vi "main.vi"() -> ()   [LabVIEW 2018]
uses:
  Module/User Event/User Event.lvlib
  Module/Message Queue/Message Queue.lvlib
  Module/Message Queue/Enqueue Message (Single).vi
  UI/TypeDefine/EnumMainDlgInit.ctl
  MainUIRef.ctl
  Module/Library-Ctrl/Library-Ctrl.lvlib
panel:
  in  "선택항목 모든버전 삭제 버튼":bool
  in  "선택항목 삭제 버튼":bool
  in  "업로드버튼":bool
  in  "업로드할 파일 정보 입력란":T1
  in  "main-lstDetailFileInfo":i32(listbox)
  in  "main-lstFileList":i32(listbox)
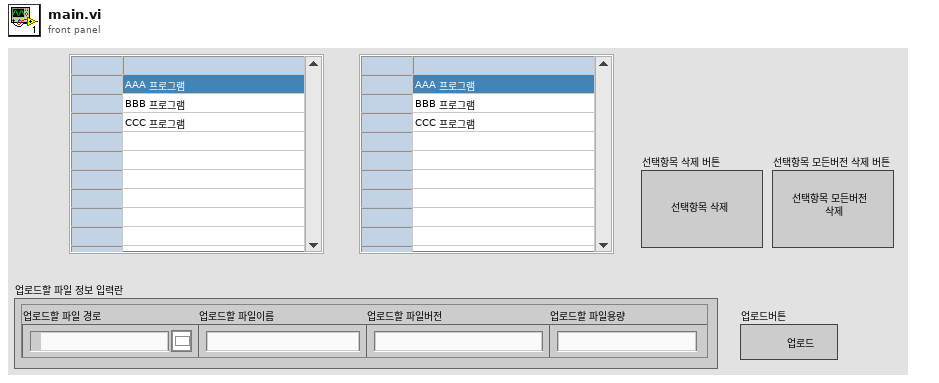
[diagram p1: front panel]
types:
  T1 = cluster{"업로드할 파일 경로":path, "업로드할 파일이름":string, "업로드할 파일버전":string, "업로드할 파일용량":string}
  T2 = typedef "MainUIRef.ctl" = cluster{"btn":cluster{"bStartBtn":refnum<vi>, "bStopBtn":refnum<vi>, "bReportBtn":refnum<vi>, "bUnitStartBtn":refnum<vi>, "bScanBtn":refnum<vi>, "bSettingBtn":refnum<vi>, "bRepeatBtn":refnum<vi>}, "status":cluster{"bEnableFailStop":refnum<vi>, "bEnableSafety":refnum<vi>, "bTestRunCheck":refnum<vi>, "bIsCompletedMaster":refnum<vi>}, "main":cluster{"lstFileList":refnum<vi>, "lstDetailFileInfo":refnum<vi>}}
  T3 = cluster{"MainUIRef":T2, "User Event":refnum<user-event>}
  T4 = cluster{"bStartBtn":refnum<vi>, "bStopBtn":refnum<vi>, "bReportBtn":refnum<vi>, "bUnitStartBtn":refnum<vi>, "bScanBtn":refnum<vi>, "bSettingBtn":refnum<vi>, "bRepeatBtn":refnum<vi>}
  T5 = cluster{"bEnableFailStop":refnum<vi>, "bEnableSafety":refnum<vi>, "bTestRunCheck":refnum<vi>, "bIsCompletedMaster":refnum<vi>}
  T6 = cluster{"lstFileList":refnum<vi>, "lstDetailFileInfo":refnum<vi>}
  T7 = typedef "Message Queue.lvlib/All Message Queues.ctl" = cluster{"UI":refnum<queue>, "Display":refnum<queue>, "Timer":refnum<queue>}
  T8 = typedef "EnumMainDlgInit.ctl" = enum16{"start", "initRef", "InitDisplayUI", "InitSetting", "InitModule", "InitOperation", "SetuipDisplayUI", "end"}
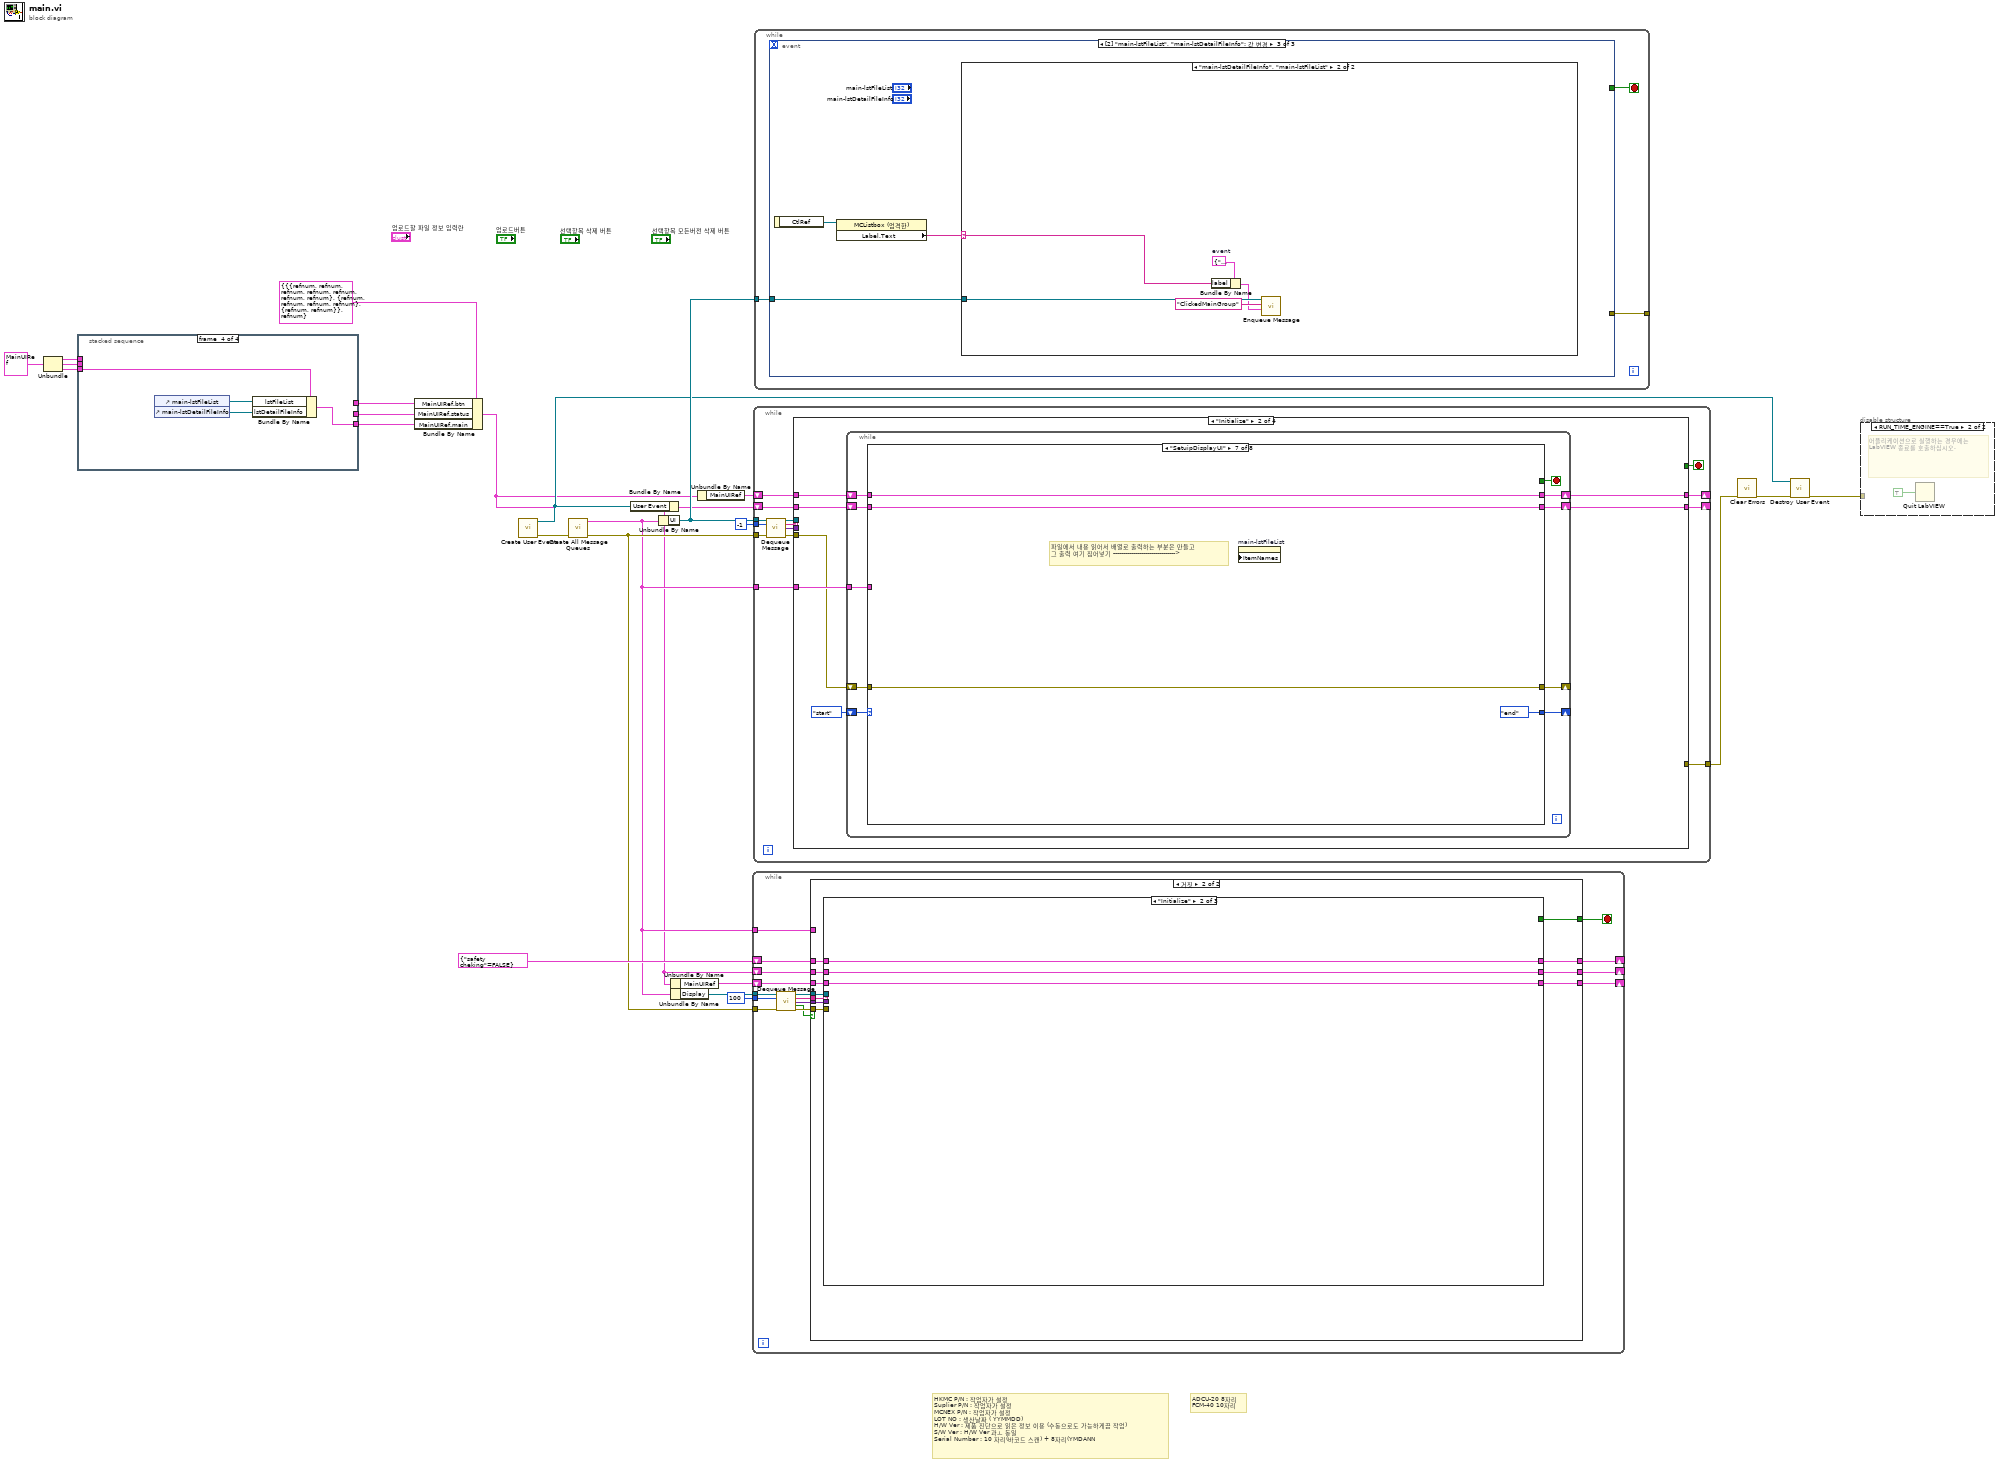
[diagram p0: block diagram]
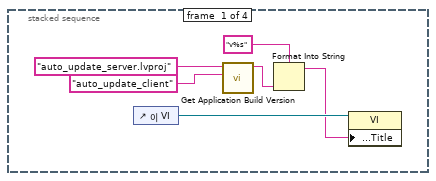
[diagram p2: hidden frame]
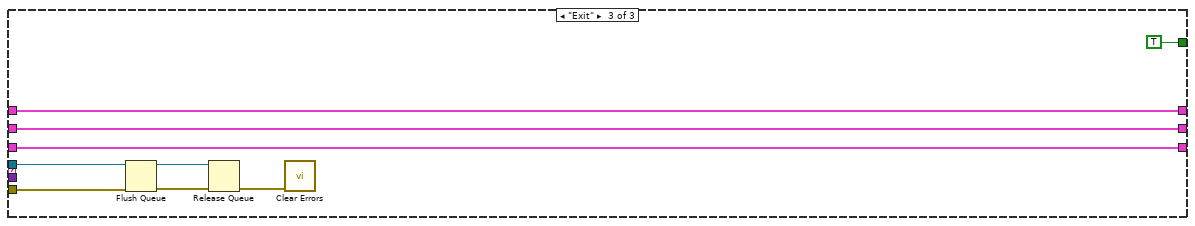
[diagram p8: hidden frame]
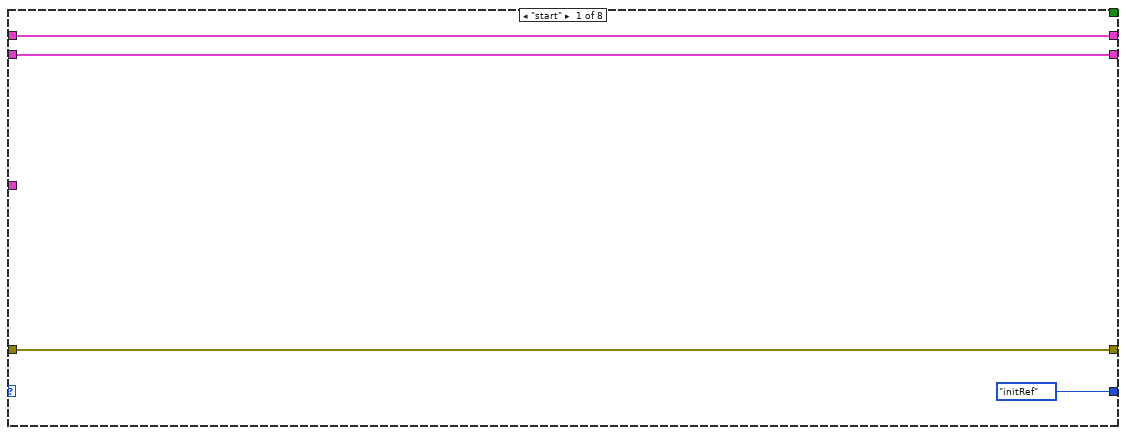
[diagram p10: hidden frame]
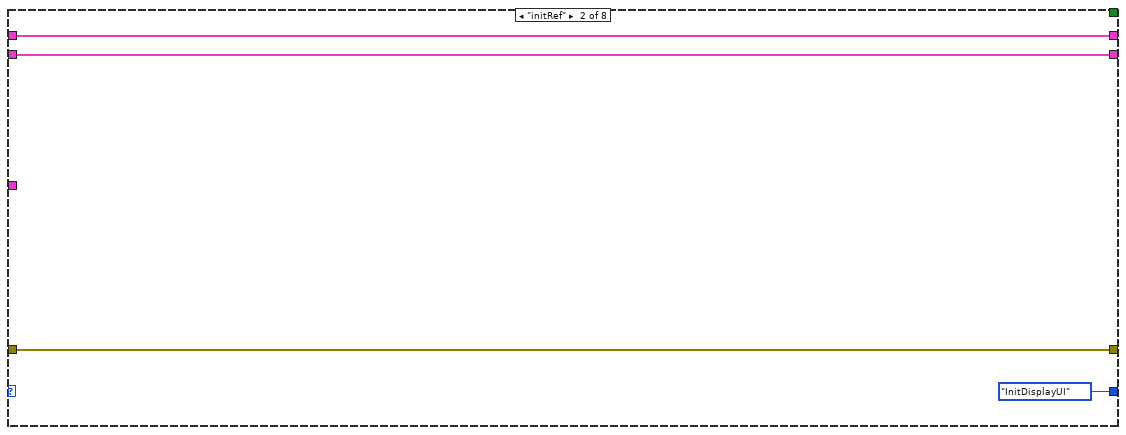
[diagram p11: hidden frame]
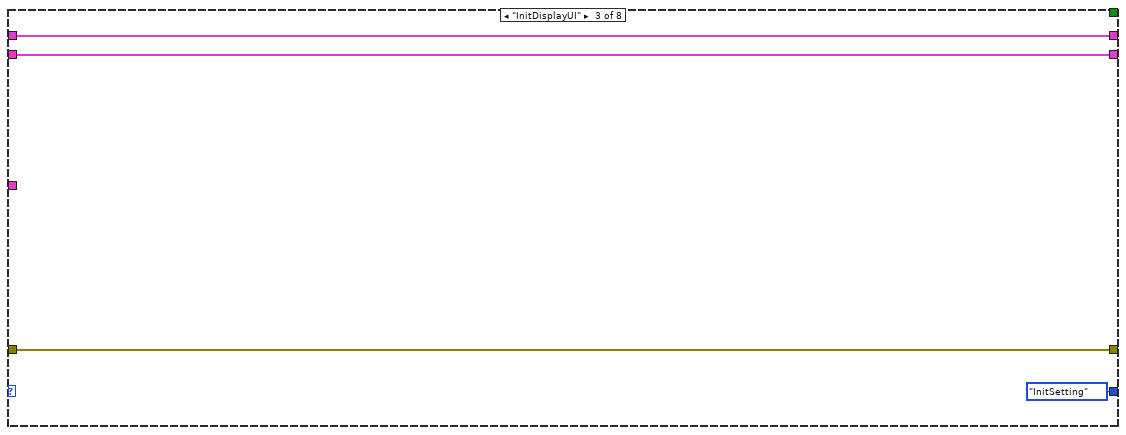
[diagram p12: hidden frame]
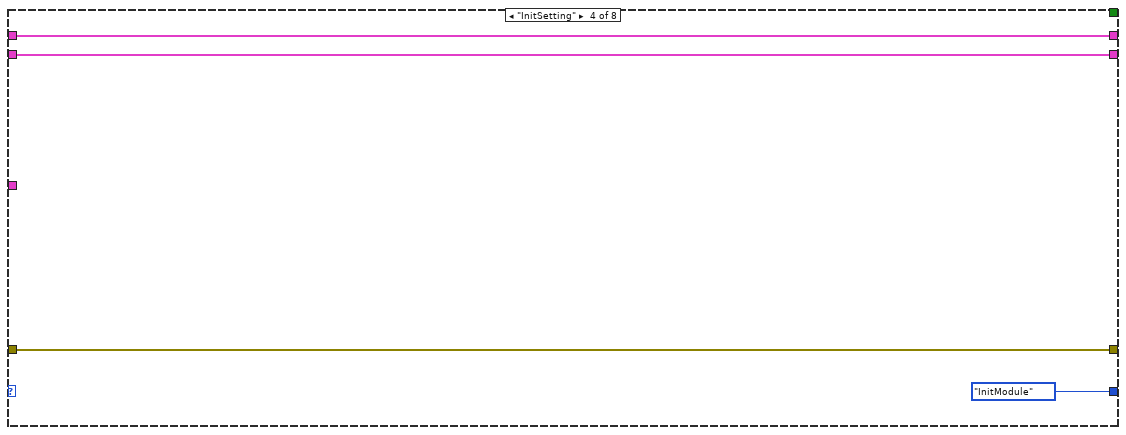
[diagram p13: hidden frame]
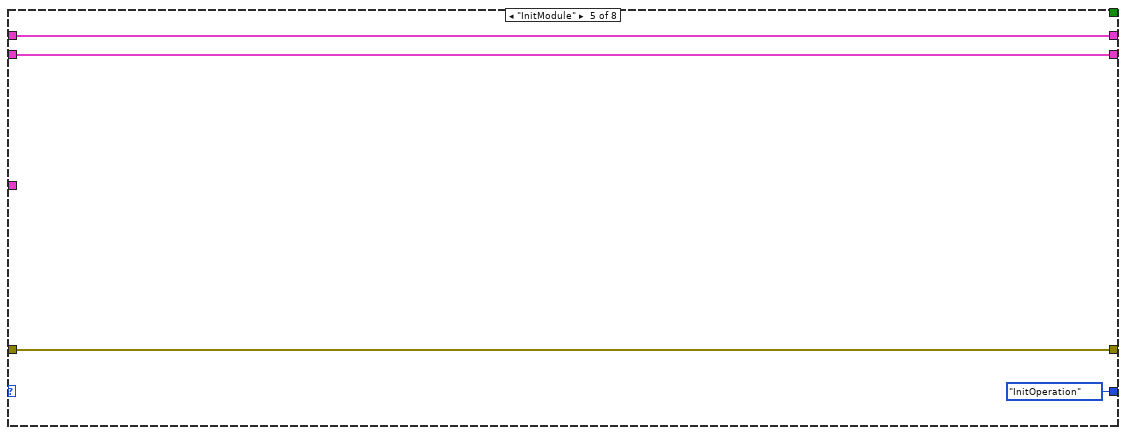
[diagram p14: hidden frame]
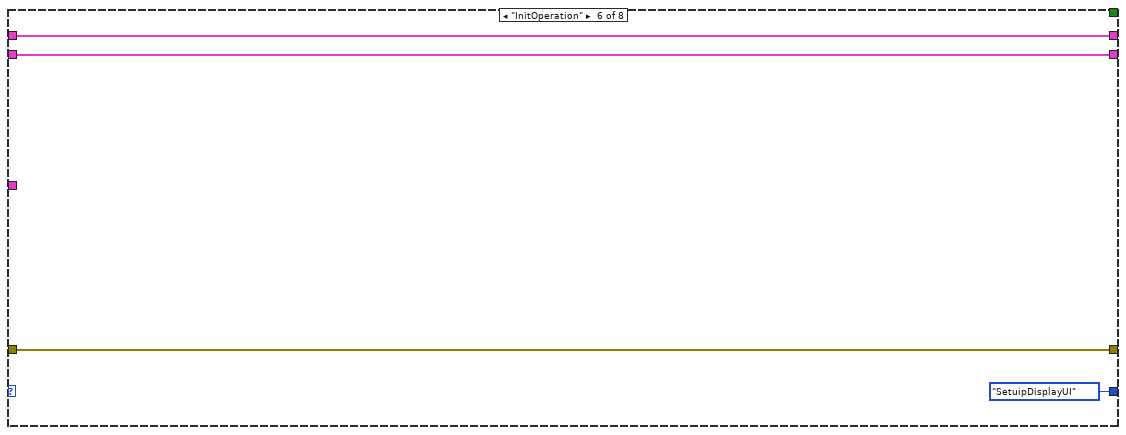
[diagram p15: hidden frame]
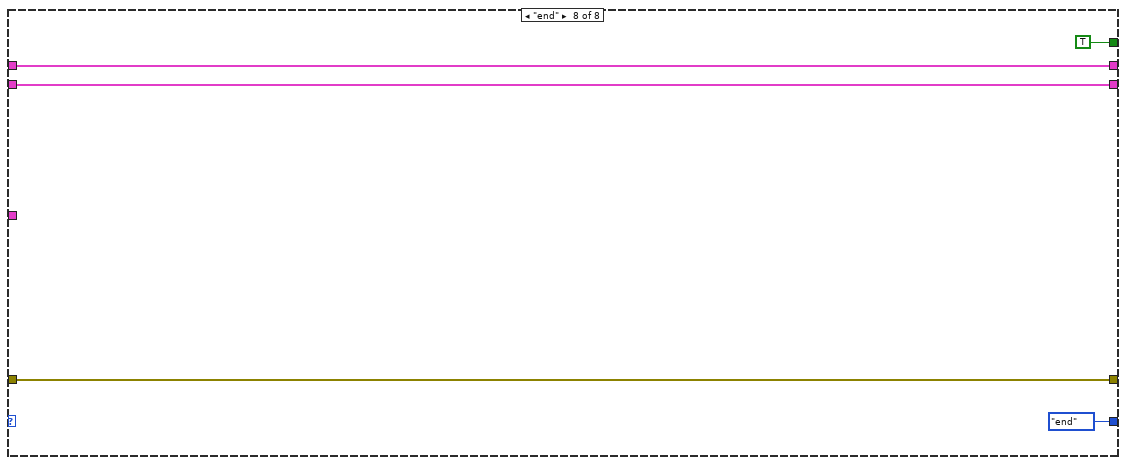
[diagram p16: hidden frame]
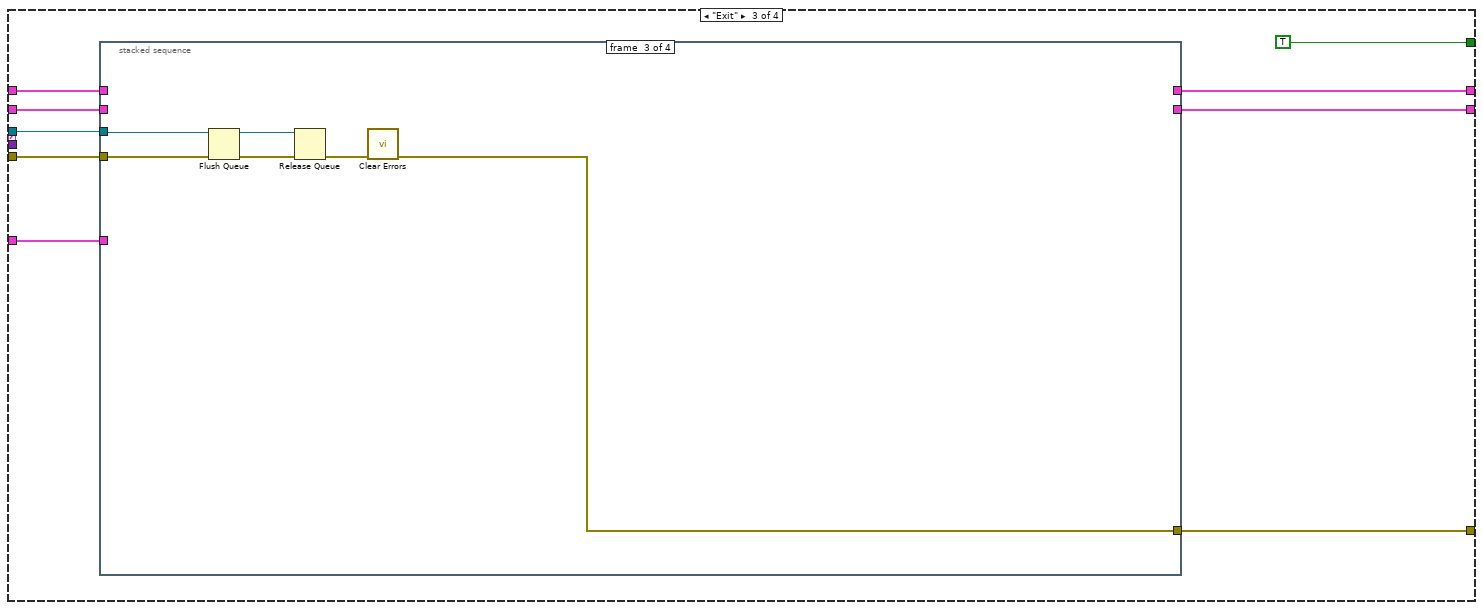
[diagram p17: hidden frame]
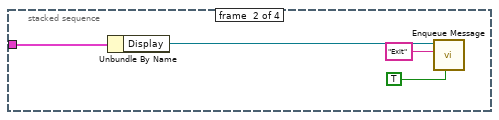
[diagram p19: hidden frame]
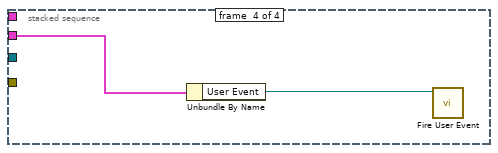
[diagram p20: hidden frame]
diagram:
  # "ADCU-20 8자리\nFCM-40 10자리"
  # "HKMC P/N : 작업자가 설정\nSuplier P/N : 작업자가 설정\nMCNEX P/N : 작업자가 설정\nLOT NO : 생산날짜 ( YYMMDD)\nH/W Ver : 제품 진단으로 읽은 정보 이용 (수동으로도 가능하게끔 작업)\nS/W Ver : H/W Ver 과ㅗ 동일\nSerial Number : 10 자리(바코드 스캔) + 8자리(YMDANN"
  n1 = Unbundle(T2 {"btn"={"bStartBtn"=refnum, "bStopBtn"=refnum, "bReportBtn"=refnum, "bUnitStartBtn"=refnum, "bScanBtn"=refnum, "bSettingBtn"=refnum, "bRepeatBtn"=refnum}, "status"={"bEnableFailStop"=refnum, "bEnableSafety"=refnum, "bTestRunCheck"=refnum, "bIsCompletedMaster"=refnum}, "main"={"lstFileList"=refnum, "lstDetailFileInfo"=refnum}} ("MainUIRef")) -> ("btn"=w10:T4, "status"=w9:T5, "main"=w8:T6)
  n2 = stacked-sequence {
    tunnel: w10 -> [_ w31 _ _]
    tunnel: w9 -> [_ _ w32 _]
    tunnel: w8 -> [_ _ _ w36]
    tunnel: [_ w31 _ _] -> w7
    tunnel: [_ _ w32 _] -> w6
    tunnel: [_ _ _ w33] -> w5
    frame #0 {
      n3 = control-ref of="이 VI"() -> (w28:refnum<vi>)
      n4 = call "Get Application Build Version.vi"("Build Specification Name"="auto_update_client", "Project Filename"="auto_update_server.lvproj") -> ("Version String"=w26:string)  [unwired: 7 in, 2 out]
      n5 = Format Into String(format string="v%s" ("포맷 문자열"), w26) -> (resulting string=w25:string)  [unwired: 2 in, 1 out]
      n6 = property class="VI"(reference=w28, "Front Panel.Title"=w25) -> ()  [unwired: 1 in, 2 out]
    }
    frame #1 {
    }
    frame #2 {
    }
    frame #3 {
      n7 = control-ref of="main-lstFileList"() -> (w35:refnum<vi>)
      n8 = control-ref of="main-lstDetailFileInfo"() -> (w34:refnum<vi>)
      n9 = Bundle By Name(cluster=w36, "lstFileList"=w35, "lstDetailFileInfo"=w34) -> (w33:T6)
    }
  }
  n10 = Bundle By Name(cluster=T3 {"MainUIRef"={"btn"={"bStartBtn"=refnum, "bStopBtn"=refnum, "bReportBtn"=refnum, "bUnitStartBtn"=refnum, "bScanBtn"=refnum, "bSettingBtn"=refnum, "bRepeatBtn"=refnum}, "status"={"bEnableFailStop"=refnum, "bEnableSafety"=refnum, "bTestRunCheck"=refnum, "bIsCompletedMaster"=refnum}, "main"={"lstFileList"=refnum, "lstDetailFileInfo"=refnum}}, "User Event"=refnum}, "MainUIRef.btn"=w7, "MainUIRef.status"=w6, "MainUIRef.main"=w5) -> (w2:T3)
  n11 = call "Create User Event.vi"() -> ("error out"=w24:errorcluster, "User Event"=w12:refnum<user-event>)  [unwired: 10 in]
  n12 = call "Create All Message Queues.vi"("error in (no error)"=w24) -> ("error out"=w14:errorcluster, "Message Queues out"=w13:T7)  [unwired: 9 in]
  n13 = Bundle By Name(cluster=w2, "User Event"=w12) -> (w4:T3)
  n14 = Unbundle By Name(w13) -> ("UI"=w23:refnum<queue>)
  n15 = Unbundle By Name(w4) -> ("MainUIRef"=w3:T2)
  n16 = Unbundle By Name(w13) -> ("Display"=w21:refnum<queue>)
  n17 = Unbundle By Name(w2) -> ("MainUIRef"=w1:T2)
  n18 = while {
    tunnel: w21 -> [w52]
    tunnel: w14 -> [w50]
    tunnel: 100 ("타임아웃(ms) (-1)") -> [w49]
    shift-right: [w42] -> _
    shift-left: w4 -> [w43]
    shift-right: [w40] -> _
    shift-left: cluster{"safety cheking":bool} {"safety cheking"=FALSE} -> [w41]
    shift-right: [w38] -> _
    shift-left: w3 -> [w39]
    tunnel: w13 -> [w37]
    stop <- w44 stop-if-true
    n19 = call "Dequeue Message.vi"("Message Queue"=w52, "타임아웃(ms) (-1)"=w49, "error in (no error)"=w50) -> ("dup Message Queue"=w51:refnum<queue>, "Message"=w45:string, "Message Data"=w48:variant, "타임아웃?"=w46:bool, "error out"=w47:errorcluster)  [unwired: 8 in]
    n20 = case shown="거짓" w46 {
      tunnel: w51 -> [_ w73]
      tunnel: w48 -> [_ w63]
      tunnel: w47 -> [_ w72]
      tunnel: w45 -> [_ w71]
      tunnel: [_ w70] -> w44
      tunnel: w43 -> [w58 w68]
      tunnel: [w56 w66] -> w42
      tunnel: w41 -> [w59 w69]
      tunnel: [w57 w67] -> w40
      tunnel: w39 -> [w55 w65]
      tunnel: [w54 w64] -> w38
      tunnel: w37 -> [w53 _]
      frame True {
        n21 = stacked-sequence {
          tunnel: w59 -> [w62]
          tunnel: w58 -> [w61]
          tunnel: [w62] -> w57
          tunnel: [w61] -> w56
          tunnel: w55 -> [w60]
          tunnel: [w60] -> w54
          tunnel: w53 -> [_]
          frame #0 {
          }
        }
      }
      frame False {
        n22 = case shown="\"Initialize\"" w71 {
          tunnel: w73 -> [_ _ w88]
          tunnel: w72 -> [_ _ w87]
          tunnel: [_ _ TRUE] -> w70
          tunnel: w69 -> [w76 w79 w82]
          tunnel: w68 -> [w75 w78 w81]
          tunnel: [w76 w79 w82] -> w67
          tunnel: [w75 w78 w81] -> w66
          tunnel: w65 -> [w74 w77 w80]
          tunnel: [w74 w77 w80] -> w64
          tunnel: w63 -> [_ _ _]
          frame Default {
          }
          frame "Initialize" {
          }
          frame "Exit" {
            n23 = Flush Queue(queue=w88, error in (no error)=w87) -> (queue out=w86:refnum<queue>, error out=w85:errorcluster)  [unwired: 1 out]
            n24 = Release Queue(queue=w86, error in (no error)=w85) -> (error out=w84:errorcluster)  [unwired: 1 in, 2 out]
            n25 = call <vilib>:"Clear Errors.vi"("error in (no error)"=w84) -> ()  [unwired: 5 in, 2 out]
          }
        }
      }
    }
  }
  n26 = while {
    tunnel: w23 -> [w102]
    tunnel: w14 -> [w100]
    tunnel: -1 ("타임아웃(ms) (-1)") -> [w99]
    tunnel: w13 -> [w94]
    shift-right: [w92] -> _
    shift-left: w1 -> [w93]
    tunnel: [w91] -> w17
    shift-right: [w89] -> _
    shift-left: w4 -> [w90]
    stop <- w95 stop-if-true
    n27 = call "Dequeue Message.vi"("Message Queue"=w102, "타임아웃(ms) (-1)"=w99, "error in (no error)"=w100) -> ("dup Message Queue"=w101:refnum<queue>, "Message"=w98:string, "Message Data"=w97:variant, "error out"=w96:errorcluster)  [unwired: 8 in, 1 out]
    n28 = case shown="\"Initialize\"" w98 {
      tunnel: w101 -> [_ _ w163 _]
      tunnel: w97 -> [_ _ _ w188]
      tunnel: w96 -> [_ w105 w162 w189]
      tunnel: [_ _ TRUE ("Priority Message? (F)") _] -> w95
      tunnel: w94 -> [_ w106 w160 w178]
      tunnel: w93 -> [w104 w111 w158 w183]
      tunnel: [w104 w109 w157 w182] -> w92
      tunnel: [_ _ w155 _] -> w91
      tunnel: w90 -> [w103 w108 w159 w181]
      tunnel: [w103 w107 w156 w180] -> w89
      frame Default {
      }
      frame "Initialize" {
        n29 = while {
          shift-right: [w119] -> w109
          shift-left: w111 -> [w120]
          shift-right: [w118] -> _
          shift-left: EnumMainDlgInit."start" ("EnumMainDlgInit") -> [w121]
          shift-right: [w115] -> w107
          shift-left: w108 -> [w116]
          tunnel: w106 -> [w114]
          shift-right: [w112] -> _
          shift-left: w105 -> [w113]
          stop <- w117 stop-if-true
          n30 = case shown="\"SetuipDisplayUI\"" w121 {
            tunnel: w120 -> [w125 w126 w132 w136 w140 w142 w147 w154]
            tunnel: [w125 w126 w132 w136 w140 w142 w147 w154] -> w119
            tunnel: [EnumMainDlgInit."initRef" ("EnumMainDlgInit") EnumMainDlgInit."InitDisplayUI" ("EnumMainDlgInit") EnumMainDlgInit."InitSetting" ("EnumMainDlgInit") EnumMainDlgInit."InitModule" ("EnumMainDlgInit") EnumMainDlgInit."InitOperation" ("EnumMainDlgInit") EnumMainDlgInit."SetuipDisplayUI" ("EnumMainDlgInit") EnumMainDlgInit."end" ("EnumMainDlgInit") EnumMainDlgInit."end" ("EnumMainDlgInit")] -> w118
            tunnel: [_ _ _ _ _ _ _ TRUE] -> w117
            tunnel: w116 -> [w122 w129 w130 w135 w139 w143 w146 w150]
            tunnel: [w122 w129 w130 w135 w139 w143 w146 w150] -> w115
            tunnel: w114 -> [_ _ _ _ _ _ _ _]
            tunnel: w113 -> [w123 w128 w131 w134 w138 w144 w148 w151]
            tunnel: [w123 w128 w131 w134 w138 w144 w148 w151] -> w112
            frame "start" {
            }
            frame "initRef" {
            }
            frame "InitDisplayUI" {
            }
            frame "InitSetting" {
            }
            frame "InitModule" {
            }
            frame "InitOperation" {
            }
            frame "SetuipDisplayUI" {
              # "파일에서 내용 읽어서 배열로 출력하는 부분은 만들고 \n그 출력 여기 집어넣기 ------------------------------->"
              n31 = property on="main-lstFileList" class="MCListbox (엄격한)" props=["ItemNames"]() -> ()  [unwired: 3 in, 2 out]
            }
            frame "end" {
            }
          }
        }
      }
      frame "Exit" {
        n32 = stacked-sequence {
          tunnel: w163 -> [_ _ w172 _]
          tunnel: w162 -> [_ _ w171 _]
          tunnel: w160 -> [_ w169 _ _]
          tunnel: [_ _ w170 _] -> w155
          tunnel: w159 -> [w164 _ _ w177]
          tunnel: w158 -> [w165 _ _ _]
          tunnel: [w165 _ _ _] -> w157
          tunnel: [w164 _ _ _] -> w156
          frame #0 {
          }
          frame #1 {
            n33 = Unbundle By Name(w169) -> ("Display"=w168:refnum<queue>)
            n34 = call-poly "Enqueue Message.vi"("Priority Message? (F)"=TRUE, "Message"="Exit", "Message Queue"=w168) -> ()  [unwired: 7 in, 2 out]
          }
          frame #2 {
            n35 = Flush Queue(queue=w172, error in (no error)=w171) -> (queue out=w175:refnum<queue>, error out=w174:errorcluster)  [unwired: 1 out]
            n36 = Release Queue(queue=w175, error in (no error)=w174) -> (error out=w173:errorcluster)  [unwired: 1 in, 2 out]
            n37 = call <vilib>:"Clear Errors.vi"("error in (no error)"=w173) -> ("error out"=w170:errorcluster)  [unwired: 5 in, 1 out]
          }
          frame #3 {
            n38 = Unbundle By Name(w177) -> ("User Event"=w176:refnum<user-event>)
            n39 = call "Fire User Event.vi"("User Event"=w176) -> ()  [unwired: 10 in, 1 out]
          }
        }
      }
      frame "ClickedMainGroup" {
        w187 = cluster{"label":string, "Data":variant} {"label"="", "Data"=variant}  # event
        n40 = Variant To Data(error in=w189, type=w187, Variant=w188) -> (data=w186:cluster{"label":string, "Data":variant}, error out=w184:errorcluster)
        n41 = Unbundle(w186) -> ("label"=w179:string, "Data"=w185:variant)
        n42 = case shown="\"main-lstFileList\"" w179 {
          tunnel: w185 -> [_ _]
          tunnel: w184 -> [_ _]
          tunnel: w183 -> [w191 w198]
          tunnel: [w191 w198] -> w182
          tunnel: w181 -> [w190 w199]
          tunnel: [w190 w199] -> w180
          tunnel: w178 -> [_ _]
          frame Default {
          }
          frame "main-lstFileList" {
            n43 = Unbundle By Name(w198) -> ("main.lstFileList"=w197:refnum<vi>)
            n44 = call "GetOneRecordFrom2DListCtrl.vi"("testcaselist in"=w197) -> ("one record"=w195:string[])  [unwired: 9 in, 1 out]
            n45 = Index Array(array=w195, index=0 ("인덱스")) -> (element=w193:string)
            n46 = Format Into String(format string="%s 가 클릭되었습니다" ("포맷 문자열"), w193) -> (resulting string=w192:string)  [unwired: 2 in, 1 out]
            n47 = One Button Dialog(message=w192) -> ()  [unwired: 1 in, 1 out]
          }
        }
      }
    }
  }
  n48 = while {
    tunnel: w23 -> [w201]
    tunnel: [w200] -> _
    stop <- w202 stop-if-true
    n49 = event shown="[2] \"main-lstFileList\", \"main-lstDetailFileInfo\": 값 변경" {
      selector: _ -> [_ _ _]
      dyn-events: _ -> [_ _ _]
      timeout: _ -> [_ _ _]
      tunnel: [_ w204 _] -> w202
      tunnel: w201 -> [_ w206 w216]
      tunnel: [_ w205 _] -> w200
      event Timeout {
        n50 = event-data() -> ()  [unwired: 1 in, 1 out]
      }
      event Panel Close? {
        n51 = event-data() -> ()  [unwired: 1 in, 4 out]
        n52 = Two Button Dialog(message="프로그램을 종료하시겠습니까?" ("메시지")) -> (T button?=w207:bool)  [unwired: 2 in]
        n53 = case shown="참" w207 {
          tunnel: w206 -> [w209 w213]
          tunnel: [w209 w212] -> _
          tunnel: [_ w211] -> w205
          tunnel: [_ TRUE] -> w204
          frame False {
          }
          frame True {
            n54 = call-poly "Enqueue Message.vi"("Priority Message? (F)"=TRUE, "Message"="Exit", "Message Queue"=w213) -> ("error out"=w211:errorcluster, "dup Message Queue"=w212:refnum<queue>)  [unwired: 7 in]
          }
        }
        n55 = event-data("Discard?"=TRUE) -> ()  [unwired: 1 in, 1 out]
      }
      event "main-lstFileList", "main-lstDetailFileInfo": Value Change {
        n56 = event-data() -> ("CtlRef"=w218:refnum<vi>)  [unwired: 1 in]
        n57 = property class="MCListbox (엄격한)"(reference=w218) -> ("Label.Text"=w217:string)  [unwired: 1 in, 2 out]
        n58 = case shown="\"main-lstDetailFileInfo\", \"main-lstFileList\"" w217 {
          selector: w217 -> [_ w221]
          tunnel: w216 -> [_ w222]
          frame Default {
          }
          frame "main-lstDetailFileInfo", "main-lstFileList" {
            w219 = cluster{"label":string, "Data":variant} {"label"="", "Data"=variant}  # event
            n59 = Bundle By Name(cluster=w219, "label"=w221) -> (w220:cluster{"label":string, "Data":variant})
            n60 = call-poly "Enqueue Message.vi"("Message Data"=w220, "Message"="ClickedMainGroup", "Message Queue"=w222) -> ()  [unwired: 7 in, 2 out]
          }
        }
      }
    }
  }
  n61 = call <vilib>:"Clear Errors.vi"("error in (no error)"=w17) -> ("error out"=w19:errorcluster)  [unwired: 5 in, 1 out]
  n62 = call "Destroy User Event.vi"("error in (no error)"=w19, "User Event"=w12) -> ("error out"=w18:errorcluster)  [unwired: 9 in]
  n63 = disable-structure "Conditional Disable Structure" shown="RUN_TIME_ENGINE==True" {
    disable-tunnel: w18 -> [_ _]
    frame condition #0 (active) {
    }
    frame condition #1 {
      # "어플리케이션으로 실행하는 경우에는 LabVIEW 종료를 호출하십시오."
      n64 = Quit LabVIEW(quit? (T)=TRUE) -> ()
    }
  }
